vi "Get Module Execution Status by ref.vi"(11 "Library":refnum<vi>) -> (0 "error out":errorcluster, 1 "Running?":bool, 2 "Status":string)   [LabVIEW 2020, in "Panter Dashboard.lvlib"]
doc: "This VI checks the Main.vi State of the selected DQMH Module"
uses:
  Panter Dashboard.lvlib
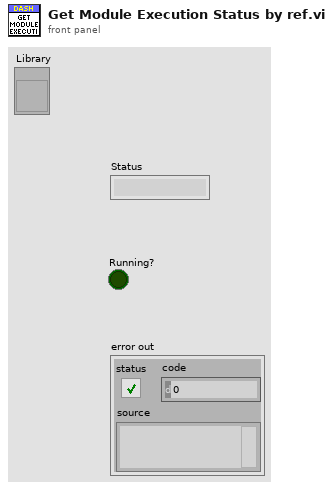
[diagram p1: front panel]
types:
  T1 = enum32{"Bad", "Idle", "Run top level", "Running"}
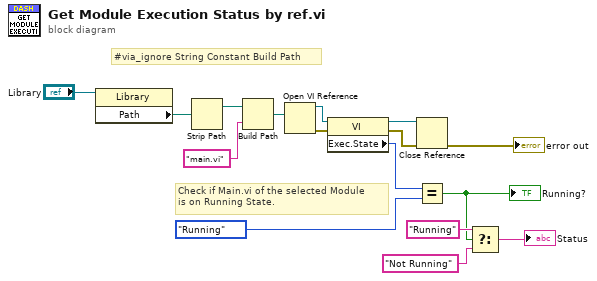
[diagram p0: block diagram]
diagram:
  # "#via_ignore String Constant Build Path"
  # "Check if Main.vi of the selected Module\nis on Running State."
  n1 = property class="Library"(reference="Library") -> ("Path"=w13:path)  [unwired: 1 in, 2 out]
  n2 = Strip Path(path=w13) -> (stripped path=w12:path)  [unwired: 1 out]
  n3 = Build Path(base path=w12, name or relative path="main.vi" ("string")) -> (appended path=w10:path)
  n4 = Open VI Reference(vi path=w10) -> (vi reference=w9:refnum<vi>, error out=w14:errorcluster)  [unwired: 5 in]
  n5 = property class="VI"(reference=w9, error in=w14) -> (reference out=w6:refnum<vi>, error out=w15:errorcluster, "Exec.State"=w8:T1)
  n6 = Close Reference(reference=w6, error in (no error)=w15) -> (error out=→"error out":errorcluster)
  n7 = Equal?(x=w8, y=T1."Running") -> (x = y?=w3:bool)
  "Running?" <- w3
  n8 = Select(t="Running", s=w3, f="Not Running") -> (s? t:f=→"Status":string)
